vi "Perspective Transform.vi"() -> ()   [LabVIEW 2018]
doc: "Perspective Transform: This is an example of a perspective transformation that maps an image from one perspective space to another. It can capture the perspective effect of objects at different depths and angles, and map it to a plane, thereby presenting a perspective effect corresponding to the real scene on the image."
uses:
  vi.lib/VIRobotics/opencv_yiku/ctls/Point2f.ctl
  vi.lib/VIRobotics/opencv_yiku/ctls/Size.ctl
  vi.lib/VIRobotics/opencv_yiku/Mat/Mat_8U/Mat_8U.lvclass
  D:/Program Files/company/National Instruments/LabVIEW 2018/vi.lib/addons/VIRobotics/opencv_yiku/Mat/Mat/Mat.lvclass
  vi.lib/VIRobotics/opencv_yiku/Cap/Cap.lvclass
  vi.lib/VIRobotics/opencv_yiku/opencv_yiku.lvlib
panel:
  out "new picture 2":picture
  in  "stop":bool
  out "new picture":picture
  # "Overview: Demonstrates how to finish Perspective Transformation.\nRequirements: Windows.\nInstructions: \n1.Make sure your computer has a camera.\n2.Run the VI"
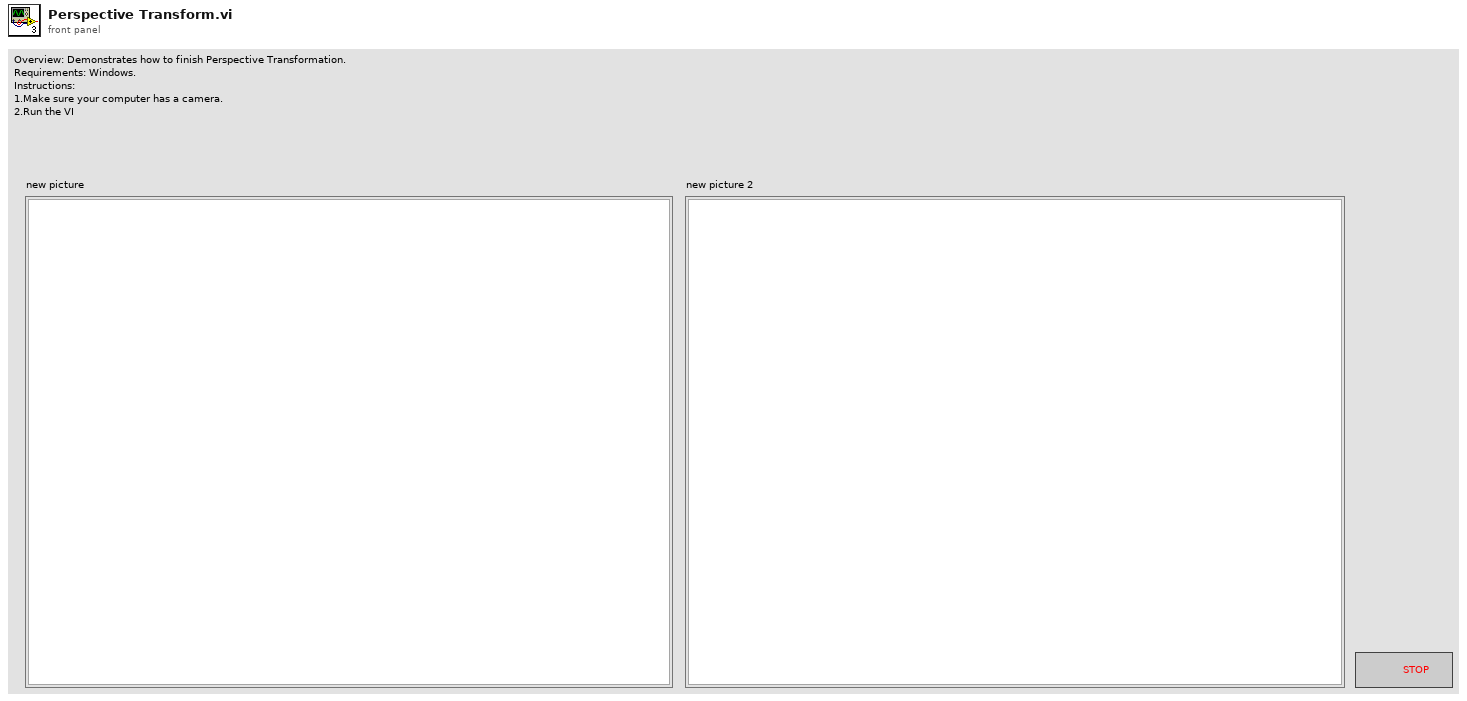
[diagram p1: front panel]
types:
  T1 = typedef "opencv_yiku.lvlib/Point2f.ctl" = cluster{"x":sgl, "y":sgl}
  T2 = typedef "opencv_yiku.lvlib/Size.ctl" = cluster{"x":i32, "y":i32}
  T3 = enum16{"COLOR_BGR2BGRA", "COLOR_BGRA2BGR", "COLOR_BGR2RGBA", "COLOR_RGBA2BGR", "COLOR_BGR2RGB", "COLOR_BGRA2RGBA", "COLOR_BGR2GRAY", "COLOR_RGB2GRAY", "COLOR_GRAY2BGR", "COLOR_GRAY2BGRA"}
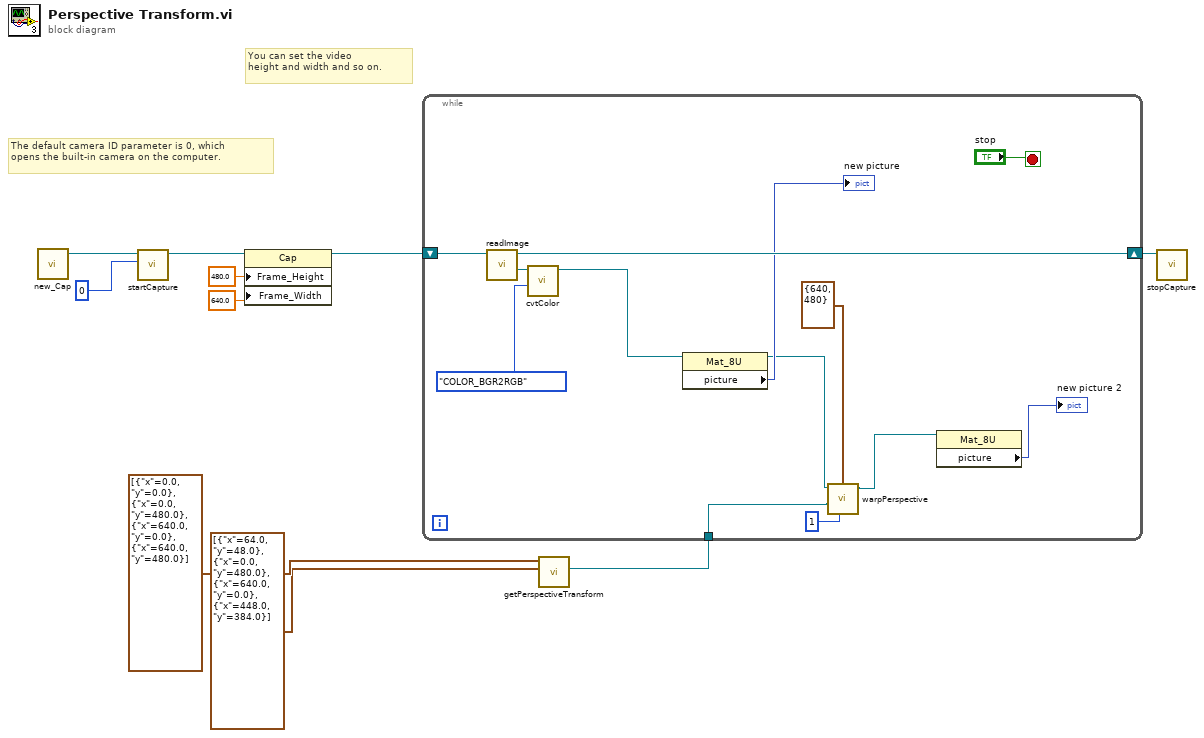
[diagram p0: block diagram]
diagram:
  # "You can set the video \nheight and width and so on."
  # "The default camera ID parameter is 0, which \nopens the built-in camera on the computer."
  n1 = call "new_Cap.vi"() -> ("Cap out"=w10:refnum<class "Cap.lvclass">)  [unwired: 10 in, 1 out]
  n2 = call "startCapture.vi"("cameraID"=0, "Cap in"=w10) -> ("Cap out"=w7:refnum<class "Cap.lvclass">)  [unwired: 8 in, 1 out]
  n3 = property class="Cap"(reference=w7, "Frame_Height"=480.0, "Frame_Width"=640.0) -> (reference out=w6:refnum<class "Cap.lvclass">)  [unwired: 1 in, 1 out]
  n4 = call "getPerspectiveTransform.vi"("dst"=T1[] [{"x"=64.0, "y"=48.0}, {"x"=0.0, "y"=480.0}, {"x"=640.0, "y"=0.0}, {"x"=448.0, "y"=384.0}] ("src"), "src"=T1[] [{"x"=0.0, "y"=0.0}, {"x"=0.0, "y"=480.0}, {"x"=640.0, "y"=0.0}, {"x"=640.0, "y"=480.0}]) -> ("M"=w1:refnum<class "Mat_32F.lvclass">)  [unwired: 8 in, 1 out]
  n5 = while {
    shift-right: [w22] -> w8
    shift-left: w6 -> [w23]
    tunnel: w1 -> [w12]
    stop <- "stop" stop-if-true
    n6 = call "readImage.vi"("Cap in"=w23) -> ("Mat out"=w20:refnum<class "Mat_8U.lvclass">, "Cap out"=w22:refnum<class "Cap.lvclass">)  [unwired: 8 in, 1 out]
    n7 = call "cvtColor.vi"("dstCn"=T3."COLOR_BGR2RGB", "src"=w20) -> ("src out"=w17:refnum<class "Mat_8U.lvclass">)  [unwired: 7 in, 2 out]
    n8 = property class="Mat_8U"(reference=w17) -> (reference out=w13:refnum<class "Mat_8U.lvclass">, "picture"=→"new picture":picture)  [unwired: 1 in, 1 out]
    n9 = call "warpPerspective.vi"("flags"=1, "Size"=T2 {"x"=640, "y"=480}, "M"=w12, "Mat in"=w13) -> ("dst out"=w15:refnum<class "Mat_8U.lvclass">)  [unwired: 6 in, 1 out]
    n10 = property class="Mat_8U"(reference=w15) -> ("picture"=→"new picture 2":picture)  [unwired: 1 in, 2 out]
  }
  n11 = call "stopCapture.vi"("Cap in"=w8) -> ()  [unwired: 10 in, 1 out]
